vi "InitFileArchive.vi"(0 "Archive In":refnum<class "Archive.lvclass">, 1 "Имя папки":string, 2 "Расширение имени файла":string, 3 "Заголовок таблицы":string[][](array[string]), 4 "Период регистрации":dbl, 5 "error in (no error)":errorcluster) -> (14 "Archive out":refnum<class "Archive.lvclass">, 19 "error out":errorcluster)   [LabVIEW 2010, in "Archive.lvclass"]
uses:
  Archive.lvclass
  Archive.lvclass/Archive.ctl
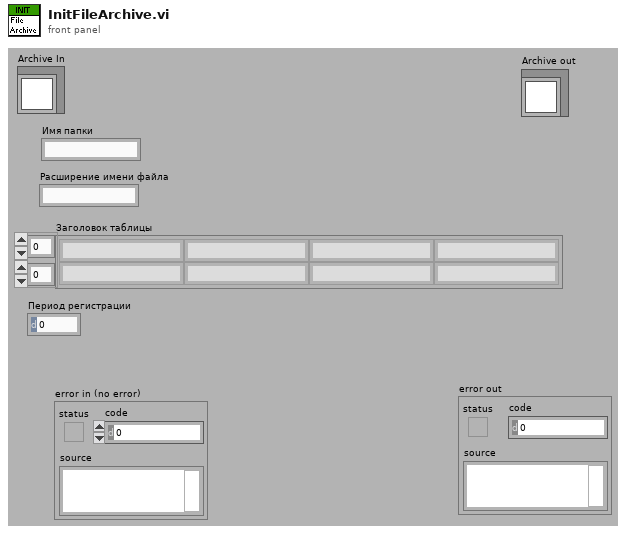
[diagram p1: front panel]
types:
  T1 = enum16{"open", "replace", "create", "open or create", "replace or create", "replace or create with confirmation"}
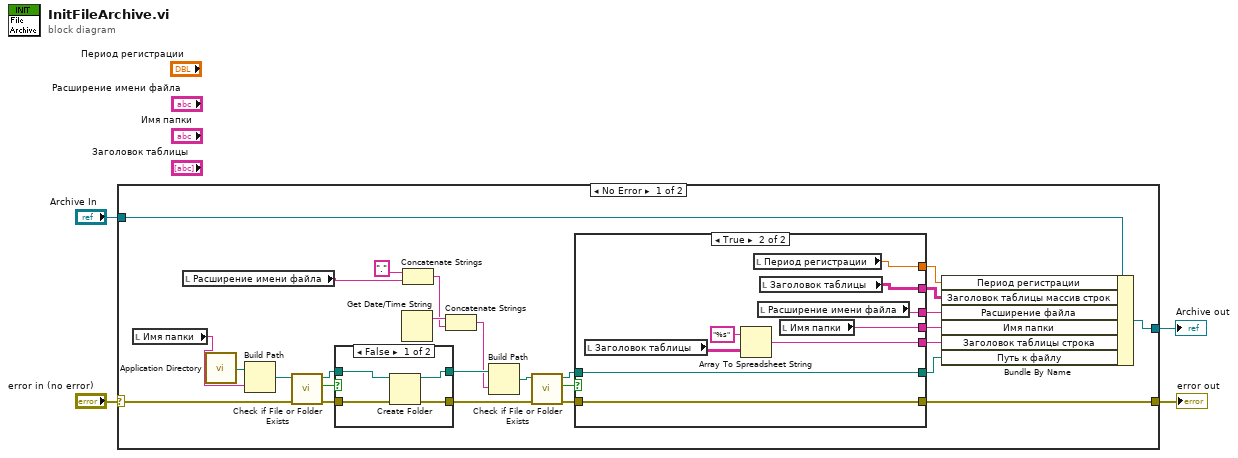
[diagram p0: block diagram]
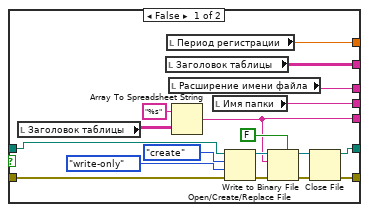
[diagram p2: hidden frame]
diagram:
  n1 = case shown="No Error" "error in (no error)" {
    selector: "error in (no error)" -> [w19 w66]
    tunnel: [w21 w66] -> w4
    tunnel: "Archive In" -> [w9 w65]
    tunnel: [w18 w65] -> w2
    frame No Error {
      n2 = local read "Имя папки"() -> (w11:string)
      n3 = local read "Расширение имени файла"() -> (w12:string)
      n4 = call <vilib>:"Application Directory.vi"() -> ("Application Directory"=w31:path)
      n5 = Build Path(base path=w31, name or relative path=w11) -> (appended path=w30:path)
      n6 = call <vilib>:"Check if File or Folder Exists.vi"("error in (no error)"=w19, "path"=w30) -> ("error out"=w25:errorcluster, "file or folder exists?"=w28:bool, "dup path"=w29:path)  [unwired: 7 in]
      n7 = case shown="False" w28 {
        tunnel: w29 -> [w62 w64]
        tunnel: [w61 w64] -> w27
        tunnel: w25 -> [w60 w63]
        tunnel: [w59 w63] -> w24
        frame False {
          n8 = Create Folder(path (use dialog)=w62, error in=w60) -> (created path=w61:path, error out=w59:errorcluster)  [unwired: 1 in, 1 out]
        }
        frame True {
        }
      }
      n9 = Get Date/Time String() -> (date string=w22:string)  [unwired: 3 in, 1 out]
      n10 = Concatenate Strings("." ("string"), w12) -> (w14:string)
      n11 = Concatenate Strings(w22, w14) -> (w26:string)
      n12 = Build Path(base path=w27, name or relative path=w26) -> (appended path=w17:path)
      n13 = call <vilib>:"Check if File or Folder Exists.vi"("error in (no error)"=w24, "path"=w17) -> ("error out"=w23:errorcluster, "file or folder exists?"=w15:bool, "dup path"=w16:path)  [unwired: 7 in]
      n14 = case shown="True" w15 {
        tunnel: w16 -> [w38 w57]
        tunnel: w23 -> [w47 w58]
        tunnel: [w40 w58] -> w21
        tunnel: [w39 w57] -> w13
        tunnel: [w36 w54] -> w10
        tunnel: [w35 w53] -> w7
        tunnel: [w34 w52] -> w8
        tunnel: [w33 w51] -> w6
        tunnel: [w32 w50] -> w5
        frame False {
          n15 = local read "Заголовок таблицы"() -> (w37:string[][])
          n16 = local read "Заголовок таблицы"() -> (w33:string[][])
          n17 = local read "Период регистрации"() -> (w32:dbl)
          n18 = local read "Расширение имени файла"() -> (w35:string)
          n19 = Array To Spreadsheet String(array=w37, 3:"%s") -> (spreadsheet string=w36:string)  [unwired: 1 in]
          n20 = local read "Имя папки"() -> (w34:string)
          n21 = Open/Create/Replace File(file path (use dialog)=w38, error in=w47, operation (0:open)=T1."create", access (0:read/write)=enum16{"read/write", "read-only", "write-only"}."write-only") -> (refnum out=w42:refnum<file>, error out=w41:errorcluster)  [unwired: 2 in, 1 out]
          n22 = Write to Binary File(file (use dialog)=w42, data=w36, error in=w41, 5:FALSE ("prepend array or string size? (T)")) -> (refnum out=w45:refnum<file>, error out=w46:errorcluster)  [unwired: 2 in, 1 out]
          n23 = Close File(refnum=w45, error in=w46) -> (path=w39:path, error out=w40:errorcluster)
        }
        frame True {
          n24 = local read "Заголовок таблицы"() -> (w55:string[][])
          n25 = Array To Spreadsheet String(array=w55, 3:"%s") -> (spreadsheet string=w54:string)  [unwired: 1 in]
          n26 = local read "Период регистрации"() -> (w50:dbl)
          n27 = local read "Расширение имени файла"() -> (w53:string)
          n28 = local read "Заголовок таблицы"() -> (w51:string[][])
          n29 = local read "Имя папки"() -> (w52:string)
        }
      }
      n30 = Bundle By Name(cluster=w9, "Период регистрации"=w5, "Заголовок таблицы массив строк"=w6, "Расширение файла"=w7, "Имя папки"=w8, "Заголовок таблицы строка"=w10, "Путь к файлу"=w13) -> (w18:refnum<class "Archive.lvclass">)
    }
    frame Error {
    }
  }
  "error out" <- w4
  "Archive out" <- w2
